vi "String.Int to Num String.vi"(8 "error in (no error)":errorcluster, 10 "Min Length (Pad with 0s)":i32=2, 11 "Int":i32) -> (0 "error out":errorcluster, 3 "Num Str":string)   [LabVIEW 2018]
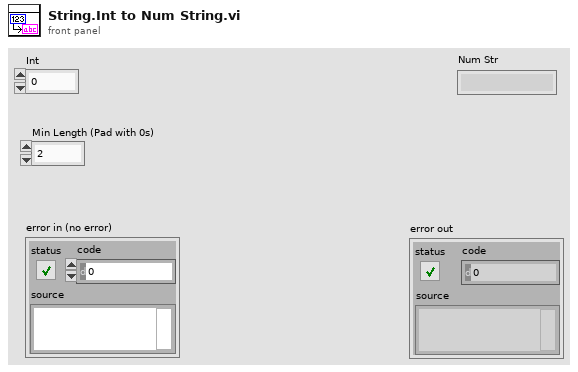
[diagram p1: front panel]
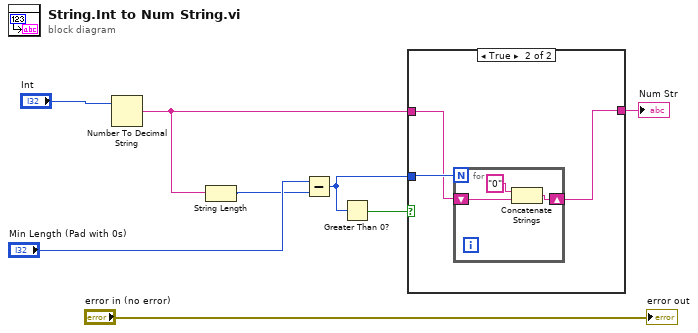
[diagram p0: block diagram]
diagram:
  n1 = Number To Decimal String(number="Int") -> (decimal integer string=w2:string)  [unwired: 1 in]
  n2 = String Length(string=w2) -> (length=w1:i32)
  n3 = Subtract(x="Min Length (Pad with 0s)", y=w1) -> (x-y=w6:i32)
  n4 = Greater Than 0?(x=w6) -> (x > 0?=w7:bool)
  n5 = case shown="True" w7 {
    tunnel: w2 -> [w9 w11]
    tunnel: w6 -> [_ w12]
    tunnel: [w9 w10] -> w5
    frame False {
    }
    frame True {
      n6 = for {
        N: w12 -> [_]
        shift-right: [w15] -> w10
        shift-left: w11 -> [w14]
        n7 = Concatenate Strings("0", w14) -> (w15:string)
      }
    }
  }
  "Num Str" <- w5
  "error out" <- "error in (no error)"
